vi "Run.vi"(8 "error in (no error)":errorcluster, 9 "Penalty":dbl, 10 "Maze (0: Empty, -1: Enemy. 1: Teammate":i32[][](array[numeric]), 11 "Runner in":refnum<class "Circle the Wagons.lvclass">) -> (0 "error out":errorcluster, 1 "Direction":T1, 2 "Action":T2, 3 "Runner out":refnum<class "Circle the Wagons.lvclass">, 4 "Replicated":refnum<class "Square.lvclass">)   [LabVIEW 2015, in "Circle the Wagons.lvclass"]
uses:
  Circle the Wagons.lvclass
  Type Defs/Action Enum.ctl
  Type Defs/Direction Enum.ctl
  Square/Square.lvclass
  DVR Cluster.ctl
  Circle the Wagons.lvclass/Circle the Wagons.ctl
  SubVIs/Read-Only Globals.vi
  Type Defs/SB Type Defs.lvlib
panel:
  # "NOTICE - YOU MUST NOT REMOVE THIS NOTICE. PER THE FOLLOWING LICENSE, YOU MAY REPRODUCE THIS SOFTWARE PROVIDED YOU FOLLOW THE TERMS\nOF THE LICENSE.\n\n---BEGIN BSD LICENSE (http://opensource.org/licenses/BSD-2-Clause)---\nCopyright (c) 2015, Endigit, Inc. <robert@endigit.com>\nAll rights reserved.\n\nRedistribution and use in source and binary forms, with or without modification, are permitted provided that the following conditions are met:\n\n1. Redistributions of source code must retain the above copyright notice, this list of conditions and the following disclaimer.\n\n2. Redistributions in binary form must reproduce the above copyright notice, this list of conditions and the following disclaimer in the documentation and/or other \nmaterials provided with the distribution.\n\nTHIS SOFTWARE IS PROVIDED BY THE COPYRIGHT HOLDERS AND CONTRIBUTORS \"AS IS\" AND ANY EXPRESS OR IMPLIED WARRANTIES, INCLUDING, BUT NOT \nLIMITED TO, THE IMPLIED WARRANTIES OF MERCHANTABILITY AND FITNESS FOR A PARTICULAR PURPOSE ARE DISCLAIMED. IN NO EVENT SHALL THE COPYRIGHT \nHOLDER OR CONTRIBUTORS BE LIABLE FOR ANY DIRECT, INDIRECT, INCIDENTAL, SPECIAL, EXEMPLARY, OR CONSEQUENTIAL DAMAGES (INCLUDING, BUT NOT \nLIMITED TO, PROCUREMENT OF SUBSTITUTE GOODS OR SERVICES; LOSS OF USE, DATA, OR PROFITS; OR BUSINESS INTERRUPTION) HOWEVER CAUSED AND ON \nANY THEORY OF LIABILITY, WHETHER IN CONTRACT, STRICT LIABILITY, OR TORT (INCLUDING NEGLIGENCE OR OTHERWISE) ARISING IN ANY WAY OUT OF THE USE \nOF THIS SOFTWARE, EVEN IF ADVISED OF THE POSSIBILITY OF SUCH DAMAGE.\n---END BSD LICENSE---"
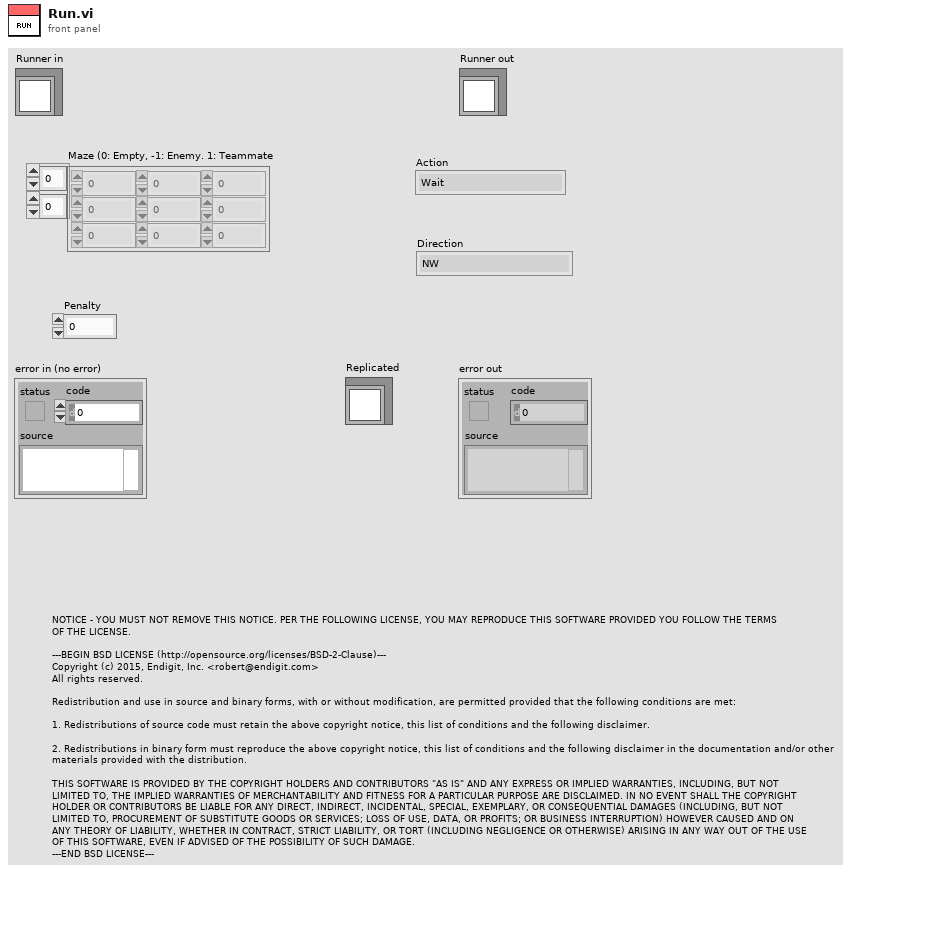
[diagram p1: front panel]
types:
  T1 = typedef "SB Type Defs.lvlib/Direction Enum.ctl" = enum16{"NW", "N", "NE", "E", "SE", "S", "SW", "W"}
  T2 = typedef "SB Type Defs.lvlib/Action Enum.ctl" = enum16{"Wait", "Move", "Attack", "Replicate"}
  T3 = typedef "Circle the Wagons.lvclass/DVR Cluster.ctl" = cluster{"Stage":i32}
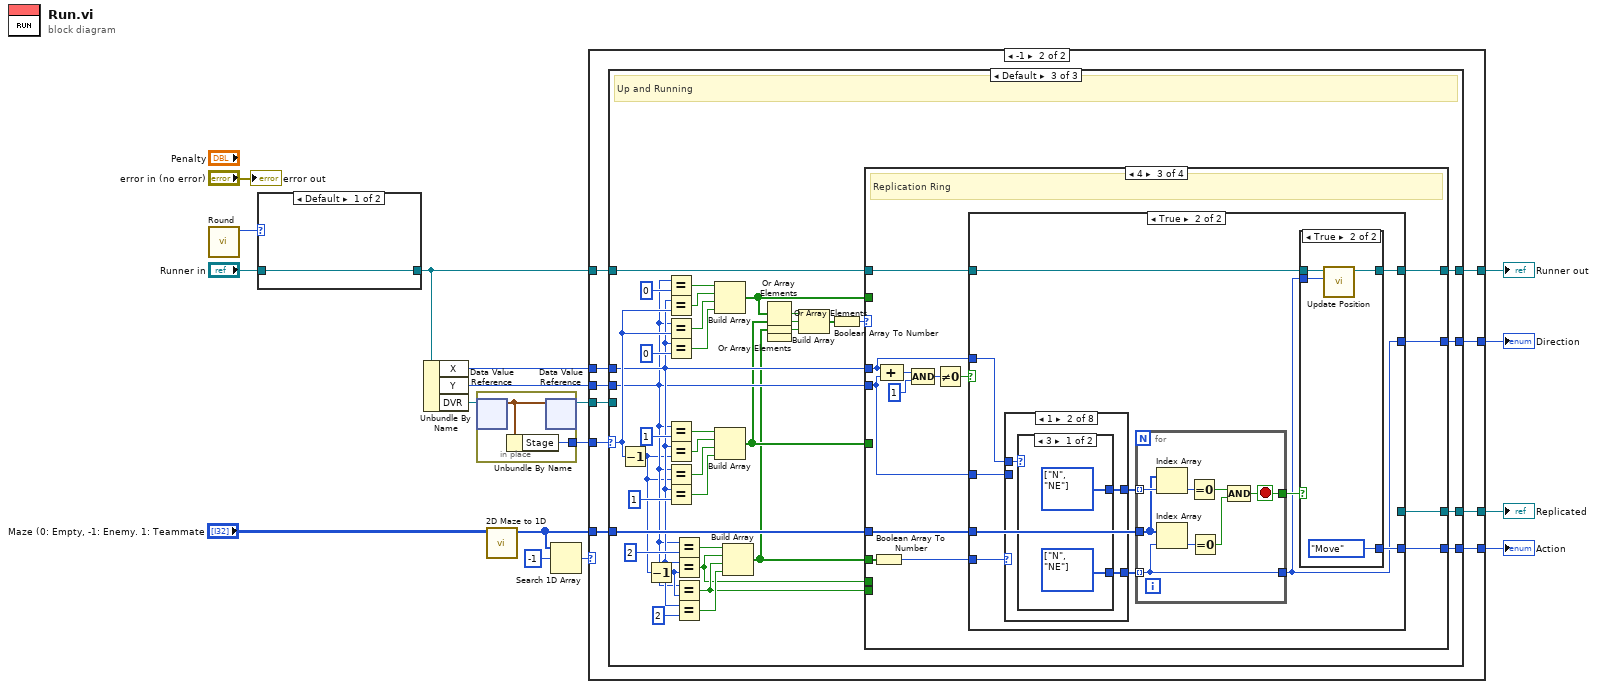
[diagram p0: block diagram]
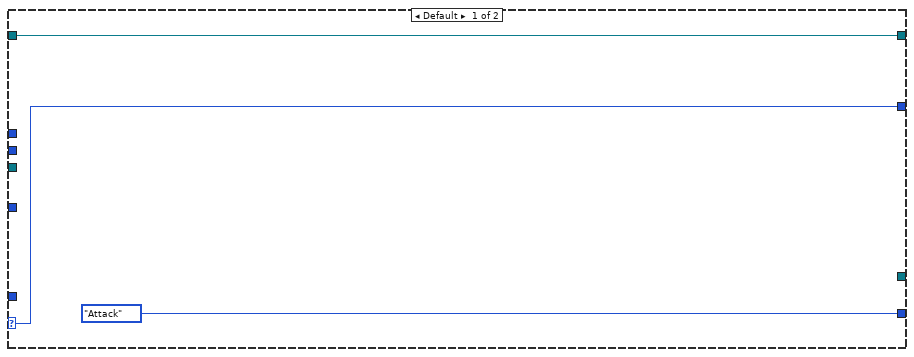
[diagram p2: hidden frame]
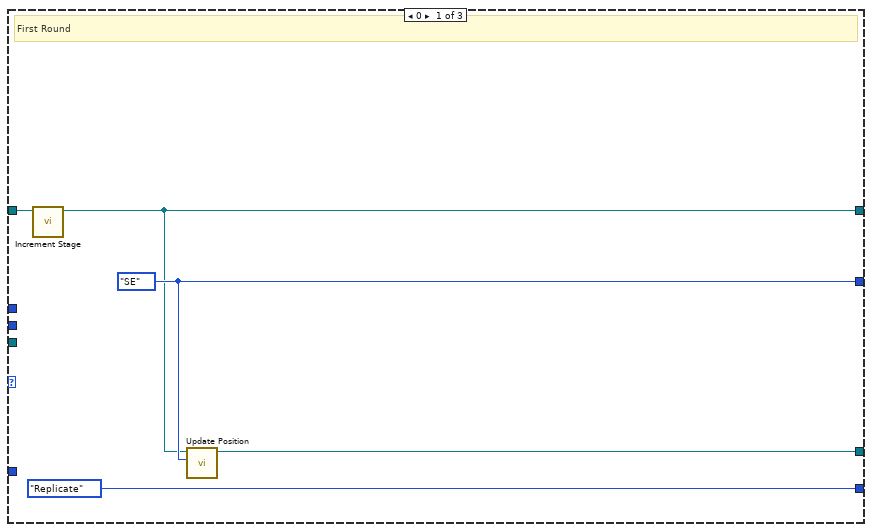
[diagram p3: hidden frame]
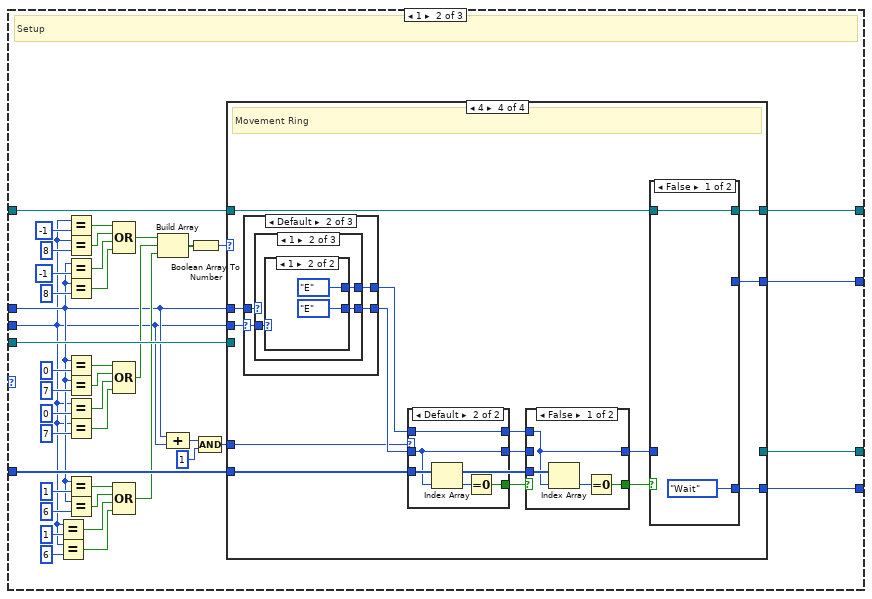
[diagram p4: hidden frame]
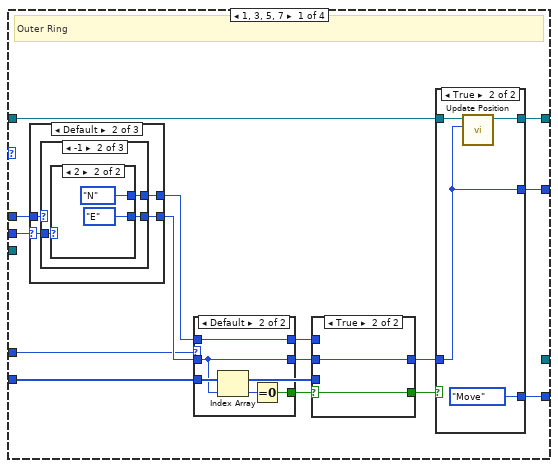
[diagram p5: hidden frame]
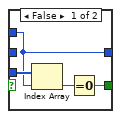
[diagram p6: hidden frame]
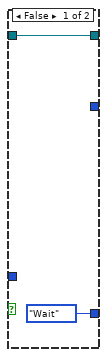
[diagram p8: hidden frame]
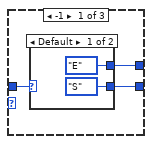
[diagram p9: hidden frame]
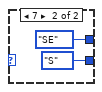
[diagram p10: hidden frame]
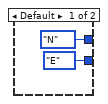
[diagram p12: hidden frame]
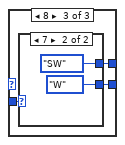
[diagram p13: hidden frame]
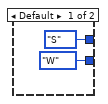
[diagram p14: hidden frame]
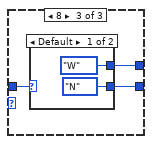
[diagram p15: hidden frame]
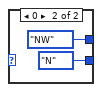
[diagram p16: hidden frame]
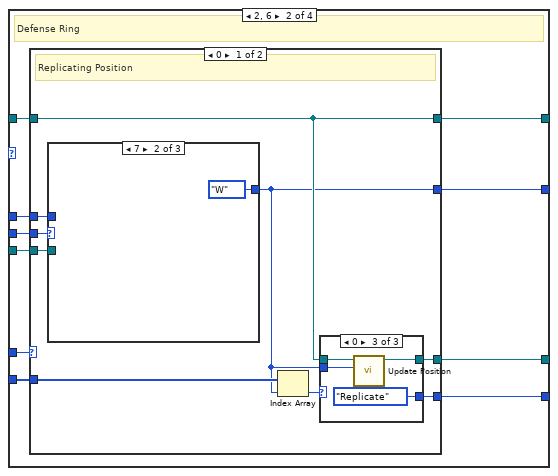
[diagram p17: hidden frame]
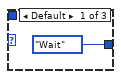
[diagram p18: hidden frame]
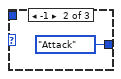
[diagram p19: hidden frame]
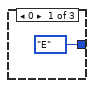
[diagram p20: hidden frame]
diagram:
  n1 = call "Round.vi"() -> ("Round"=w16:i32)  [unwired: 11 in]
  n2 = case shown="Default" w16 {
    tunnel: "Runner in" -> [w18 w21]
    tunnel: [w18 w19] -> w13
    frame Default {
    }
    frame 0 {
      n3 = New Data Value Reference(data value=T3 {"Stage"=0} ("DVR Cluster")) -> (data value reference=w20:refnum<data-value>)  [unwired: 1 in, 1 out]
      n4 = Bundle By Name(cluster=w21, "DVR"=w20) -> (w19:refnum<class "Circle the Wagons.lvclass">)
    }
  }
  n5 = Unbundle By Name(w13) -> ("X"=w11:i32, "Y"=w10:i32, "DVR"=w14:refnum<data-value>)
  n6 = in-place {
    in-place-border: [w23] -> w9
    n7 = in-place-dvr #1(w14) -> (w24:T3)  [unwired: 1 out]
    n8 = Unbundle By Name(w24) -> ("Stage"=w23:i32)
    n9 = in-place-dvr #1(w24) -> (w4:refnum<data-value>)  [unwired: 1 out]
  }
  n10 = call "2D Maze to 1D.vi"("Maze (0: Empty, -1: Enemy. >0: Teammate"="Maze (0: Empty, -1: Enemy. 1: Teammate") -> ("1D Maze"=w2:i32[])  [unwired: 10 in]
  n11 = Search 1D Array(1D array=w2, element=-1) -> (index of element=w1:i32)  [unwired: 1 in]
  n12 = case shown="-1" w1 {
    selector: w1 -> [w25 _]
    tunnel: w13 -> [w27 w37]
    tunnel: [w27 w36] -> w12
    tunnel: w11 -> [_ w35]
    tunnel: w10 -> [_ w34]
    tunnel: w9 -> [_ w33]
    tunnel: [w25 w32] -> w8
    tunnel: [Action_Enum."Attack" ("Action") w31] -> w7
    tunnel: [_ w30] -> w6
    tunnel: w4 -> [_ w29]
    tunnel: w2 -> [_ w28]
    frame Default {
    }
    frame -1 {
      n13 = case shown="Default" w33 {
        selector: w33 -> [_ _ w369]
        tunnel: w37 -> [w41 w82 w381]
        tunnel: [w38 w77 w377] -> w36
        tunnel: w35 -> [_ w45 w355]
        tunnel: w34 -> [_ w44 w354]
        tunnel: w28 -> [_ w83 w382]
        tunnel: [w40 w81 w380] -> w32
        tunnel: [Action_Enum."Replicate" ("Action") w80 w379] -> w31
        tunnel: w29 -> [_ w79 _]
        tunnel: [w39 w78 w378] -> w30
        frame 0 {
          w40 = Direction_Enum."SE" ("Direction")
          # "First Round"
          n14 = call "Increment Stage.vi"("Circle the Wagons in"=w41) -> ("Circle the Wagons out"=w38:refnum<class "Circle the Wagons.lvclass">)  [unwired: 10 in]
          n15 = call "Update Position.vi"("Direction"=w40, "Circle the Wagons in"=w38) -> ("Circle the Wagons out"=w39:refnum<class "Circle the Wagons.lvclass">)  [unwired: 9 in]
        }
        frame 1 {
          # "Setup"
          n16 = Equal?(x=w44, y=1) -> (x = y?=w56:bool)
          n17 = Equal?(x=w44, y=6) -> (x = y?=w55:bool)
          n18 = Equal?(x=w44, y=-1) -> (x = y?=w65:bool)
          n19 = Equal?(x=w44, y=8) -> (x = y?=w66:bool)
          n20 = Equal?(x=w45, y=-1) -> (x = y?=w68:bool)
          n21 = Equal?(x=w45, y=8) -> (x = y?=w67:bool)
          n22 = Equal?(x=w45, y=0) -> (x = y?=w72:bool)
          n23 = Equal?(x=w45, y=7) -> (x = y?=w71:bool)
          n24 = Equal?(x=w44, y=0) -> (x = y?=w69:bool)
          n25 = Equal?(x=w44, y=7) -> (x = y?=w70:bool)
          n26 = Equal?(x=w45, y=1) -> (x = y?=w53:bool)
          n27 = Equal?(x=w45, y=6) -> (x = y?=w54:bool)
          n28 = Compound Arithmetic op=OR(w65, w66, w68, w67) -> (w60:bool)
          n29 = Compound Arithmetic op=OR(w72, w71, w69, w70) -> (w59:bool)
          n30 = Compound Arithmetic op=OR(w53, w54, w56, w55) -> (w48:bool)
          n31 = Build Array(w60, w59, w48) -> (w58:bool[])
          n32 = Compound Arithmetic op=ADD(w45, w44) -> (w46:i32)
          n33 = Boolean Array To Number(Boolean array=w58) -> (number=w57:u32)
          n34 = Compound Arithmetic op=AND(w46, 1 ("value")) -> (w43:i32)
          n35 = case shown="4" w57 {
            tunnel: w83 -> [w92 w152 w221 w288]
            tunnel: w82 -> [w98 w159 w228 w294]
            tunnel: [w97 w158 w227 w293] -> w81
            tunnel: [w96 w157 w226 w292] -> w80
            tunnel: w79 -> [_ w150 _ _]
            tunnel: [_ w156 w225 _] -> w78
            tunnel: [w95 w155 w224 w291] -> w77
            tunnel: w45 -> [w94 w154 w223 w290]
            tunnel: w44 -> [w93 w153 w222 w289]
            tunnel: w43 -> [w84 w151 w220 w280]
            frame 1, 3, 5, 7 {
              # "Outer Ring"
              n36 = case shown="Default" w93 {
                selector: w93 -> [_ w125 _]
                tunnel: w94 -> [w119 w127 w144]
                tunnel: [w120 w128 w145] -> w90
                tunnel: [w118 w126 w143] -> w91
                frame -1 {
                  n37 = case shown="Default" w119 {
                    tunnel: [Direction_Enum."E" ("Direction") Direction_Enum."SE" ("Direction")] -> w120
                    tunnel: [Direction_Enum."S" ("Direction") Direction_Enum."S" ("Direction")] -> w118
                    frame Default {
                    }
                    frame 7 {
                    }
                  }
                }
                frame Default {
                  n38 = case shown="-1" w127 {
                    tunnel: [_ w131 w138] -> w128
                    tunnel: [_ w130 w137] -> w126
                    tunnel: w125 -> [_ w129 w136]
                    frame Default {
                    }
                    frame -1 {
                      n39 = case shown="2" w129 {
                        tunnel: [Direction_Enum."N" ("Direction") Direction_Enum."N" ("Direction")] -> w131
                        tunnel: [Direction_Enum."E" ("Direction") Direction_Enum."E" ("Direction")] -> w130
                        frame Default {
                        }
                        frame 2 {
                        }
                      }
                    }
                    frame 8 {
                      n40 = case shown="7" w136 {
                        tunnel: [Direction_Enum."S" ("Direction") Direction_Enum."SW" ("Direction")] -> w138
                        tunnel: [Direction_Enum."W" ("Direction") Direction_Enum."W" ("Direction")] -> w137
                        frame Default {
                        }
                        frame 7 {
                        }
                      }
                    }
                  }
                }
                frame 8 {
                  n41 = case shown="Default" w144 {
                    tunnel: [Direction_Enum."W" ("Direction") Direction_Enum."NW" ("Direction")] -> w145
                    tunnel: [Direction_Enum."N" ("Direction") Direction_Enum."N" ("Direction")] -> w143
                    frame Default {
                    }
                    frame 0 {
                    }
                  }
                }
              }
              n42 = case shown="Default" w84 {
                tunnel: w92 -> [_ w111]
                tunnel: w91 -> [w105 w107]
                tunnel: [_ w109] -> w89
                tunnel: w90 -> [w106 w108]
                tunnel: [w106 w108] -> w88
                tunnel: [w105 w107] -> w87
                frame 0 {
                }
                frame Default {
                  n43 = Index Array(array=w111, index=w107) -> (element=w110:i32)
                  n44 = Equal To 0?(x=w110) -> (x = 0?=w109:bool)
                }
              }
              n45 = case shown="True" w89 {
                selector: w89 -> [_ w103]
                tunnel: w88 -> [w99 _]
                tunnel: w87 -> [_ w104]
                tunnel: [w99 w104] -> w85
                tunnel: [w100 w103] -> w86
                tunnel: w92 -> [w102 _]
                frame False {
                  n46 = Index Array(array=w102, index=w99) -> (element=w101:i32)
                  n47 = Equal To 0?(x=w101) -> (x = 0?=w100:bool)
                }
                frame True {
                }
              }
              n48 = case shown="True" w86 {
                tunnel: w98 -> [w113 w117]
                tunnel: [w113 w116] -> w95
                tunnel: [Action_Enum."Wait" ("Action") Action_Enum."Move" ("Action")] -> w96
                tunnel: [_ w114] -> w97
                tunnel: w85 -> [_ w114]
                frame False {
                }
                frame True {
                  n49 = call "Update Position.vi"("Direction"=w114, "Circle the Wagons in"=w117) -> ("Circle the Wagons out"=w116:refnum<class "Circle the Wagons.lvclass">)  [unwired: 9 in]
                }
              }
            }
            frame 2, 6 {
              # "Defense Ring"
              n50 = case shown="0" w151 {
                tunnel: w154 -> [w167 w200]
                tunnel: w153 -> [w166 w199]
                tunnel: w152 -> [w168 w196]
                tunnel: w159 -> [w162 w198]
                tunnel: [w161 w202] -> w158
                tunnel: [w164 w201] -> w157
                tunnel: [w163 _] -> w156
                tunnel: [w162 w197] -> w155
                tunnel: w150 -> [w160 _]
                frame 0 {
                  # "Replicating Position"
                  n51 = case shown="7" w166 {
                    selector: w166 -> [_ _ w178]
                    tunnel: w167 -> [_ _ w180]
                    tunnel: [Direction_Enum."E" ("Direction") Direction_Enum."W" ("Direction") w179] -> w161
                    tunnel: w160 -> [_ _ w177]
                    frame 0 {
                    }
                    frame 7 {
                    }
                    frame Default {
                      n52 = case shown="7" w180 {
                        tunnel: [_ Direction_Enum."N" ("Direction") Direction_Enum."S" ("Direction")] -> w179
                        tunnel: w178 -> [_ w182 _]
                        tunnel: w177 -> [_ w181 _]
                        frame Default {
                        }
                        frame 0 {
                          n53 = case shown="2" w182 {
                            tunnel: w181 -> [_ w184]
                            frame Default {
                            }
                            frame 2 {
                              n54 = in-place {
                                n55 = in-place-dvr #2(w184) -> (w187:T3)  [unwired: 1 out]
                                n56 = Bundle By Name(cluster=w187, "Stage"=7) -> (w185:T3)
                                n57 = in-place-dvr #2(w185) -> ()  [unwired: 2 out]
                              }
                            }
                          }
                        }
                        frame 7 {
                        }
                      }
                    }
                  }
                  n58 = Index Array(array=w168, index=w161) -> (element=w165:i32)
                  n59 = case shown="0" w165 {
                    tunnel: [Action_Enum."Wait" ("Action") Action_Enum."Attack" ("Action") Action_Enum."Replicate" ("Action")] -> w164
                    tunnel: [_ _ w173] -> w163
                    tunnel: w161 -> [_ _ w172]
                    tunnel: w162 -> [_ _ w171]
                    frame Default {
                    }
                    frame -1 {
                    }
                    frame 0 {
                      n60 = call "Update Position.vi"("Direction"=w172, "Circle the Wagons in"=w171) -> ("Circle the Wagons out"=w173:refnum<class "Circle the Wagons.lvclass">)  [unwired: 9 in]
                    }
                  }
                }
                frame Default {
                  # "Non-replicating Position"
                  n61 = case shown="0" w200 {
                    tunnel: [Direction_Enum."W" ("Direction") Direction_Enum."E" ("Direction") w215] -> w194
                    tunnel: [Direction_Enum."NW" ("Direction") Direction_Enum."SE" ("Direction") w214] -> w189
                    tunnel: w199 -> [_ _ w213]
                    frame 0 {
                    }
                    frame 7 {
                    }
                    frame Default {
                      n62 = case shown="7" w213 {
                        tunnel: [_ Direction_Enum."N" ("Direction") Direction_Enum."S" ("Direction")] -> w215
                        tunnel: [_ Direction_Enum."NE" ("Direction") Direction_Enum."SW" ("Direction")] -> w214
                        frame Default {
                        }
                        frame 0 {
                        }
                        frame 7 {
                        }
                      }
                    }
                  }
                  n63 = Index Array(array=w196, index=w189) -> (element=w195:i32)
                  n64 = Index Array(array=w196, index=w194) -> (element=w193:i32)
                  n65 = Equal To 0?(x=w193) -> (x = 0?=w191:bool)
                  n66 = Equal To 0?(x=w195) -> (x = 0?=w192:bool)
                  n67 = Compound Arithmetic op=AND(w192, w191) -> (w190:bool)
                  n68 = case shown="True" w190 {
                    tunnel: w198 -> [w204 w208]
                    tunnel: [w204 w207] -> w197
                    tunnel: [Action_Enum."Wait" ("Action") Action_Enum."Move" ("Action")] -> w201
                    tunnel: [_ w205] -> w202
                    tunnel: w189 -> [_ w205]
                    frame False {
                    }
                    frame True {
                      n69 = call "Update Position.vi"("Direction"=w205, "Circle the Wagons in"=w208) -> ("Circle the Wagons out"=w207:refnum<class "Circle the Wagons.lvclass">)  [unwired: 9 in]
                    }
                  }
                }
              }
            }
            frame Default {
              # "Replication Ring"
              n70 = case shown="0" w220 {
                tunnel: w223 -> [w232 w260]
                tunnel: w222 -> [w231 w259]
                tunnel: w221 -> [w236 w256]
                tunnel: w228 -> [w229 w258]
                tunnel: [w230 w262] -> w227
                tunnel: [w234 w261] -> w226
                tunnel: [w233 _] -> w225
                tunnel: [w229 w257] -> w224
                frame 0 {
                  # "Replicating Position"
                  n71 = case shown="2" w231 {
                    tunnel: w232 -> [_ _ w246]
                    tunnel: [Direction_Enum."E" ("Direction") Direction_Enum."W" ("Direction") w245] -> w230
                    frame 2 {
                    }
                    frame 5 {
                    }
                    frame Default {
                      n72 = case shown="5" w246 {
                        tunnel: [_ Direction_Enum."N" ("Direction") Direction_Enum."S" ("Direction")] -> w245
                        frame Default {
                        }
                        frame 2 {
                        }
                        frame 5 {
                        }
                      }
                    }
                  }
                  n73 = Index Array(array=w236, index=w230) -> (element=w235:i32)
                  n74 = case shown="0" w235 {
                    tunnel: [Action_Enum."Wait" ("Action") Action_Enum."Attack" ("Action") Action_Enum."Replicate" ("Action")] -> w234
                    tunnel: [_ _ w241] -> w233
                    tunnel: w230 -> [_ _ w240]
                    tunnel: w229 -> [_ _ w239]
                    frame Default {
                    }
                    frame -1 {
                    }
                    frame 0 {
                      n75 = call "Update Position.vi"("Direction"=w240, "Circle the Wagons in"=w239) -> ("Circle the Wagons out"=w241:refnum<class "Circle the Wagons.lvclass">)  [unwired: 9 in]
                    }
                  }
                }
                frame Default {
                  # "Non-replicating Position"
                  n76 = case shown="Default" w260 {
                    tunnel: [Direction_Enum."W" ("Direction") Direction_Enum."E" ("Direction") w275] -> w254
                    tunnel: [Direction_Enum."NW" ("Direction") Direction_Enum."SE" ("Direction") w274] -> w249
                    tunnel: w259 -> [_ _ w273]
                    frame 2 {
                    }
                    frame 5 {
                    }
                    frame Default {
                      n77 = case shown="2" w273 {
                        tunnel: [_ Direction_Enum."N" ("Direction") Direction_Enum."S" ("Direction")] -> w275
                        tunnel: [_ Direction_Enum."NE" ("Direction") Direction_Enum."SW" ("Direction")] -> w274
                        frame Default {
                        }
                        frame 2 {
                        }
                        frame 5 {
                        }
                      }
                    }
                  }
                  n78 = Index Array(array=w256, index=w249) -> (element=w255:i32)
                  n79 = Index Array(array=w256, index=w254) -> (element=w253:i32)
                  n80 = Equal To 0?(x=w253) -> (x = 0?=w251:bool)
                  n81 = Equal To 0?(x=w255) -> (x = 0?=w252:bool)
                  n82 = Compound Arithmetic op=AND(w252, w251) -> (w250:bool)
                  n83 = case shown="True" w250 {
                    tunnel: w258 -> [w264 w268]
                    tunnel: [w264 w267] -> w257
                    tunnel: [Action_Enum."Wait" ("Action") Action_Enum."Move" ("Action")] -> w261
                    tunnel: [_ w265] -> w262
                    tunnel: w249 -> [_ w265]
                    frame False {
                    }
                    frame True {
                      n84 = call "Update Position.vi"("Direction"=w265, "Circle the Wagons in"=w268) -> ("Circle the Wagons out"=w267:refnum<class "Circle the Wagons.lvclass">)  [unwired: 9 in]
                    }
                  }
                }
              }
            }
            frame 4 {
              # "Movement Ring"
              n85 = case shown="Default" w289 {
                selector: w289 -> [_ w321 _]
                tunnel: w290 -> [w315 w323 w340]
                tunnel: [w316 w324 w341] -> w286
                tunnel: [w314 w322 w339] -> w287
                frame 1 {
                  n86 = case shown="Default" w315 {
                    tunnel: [Direction_Enum."E" ("Direction") Direction_Enum."S" ("Direction")] -> w316
                    tunnel: [Direction_Enum."S" ("Direction") Direction_Enum."S" ("Direction")] -> w314
                    frame Default {
                    }
                    frame 6 {
                    }
                  }
                }
                frame Default {
                  n87 = case shown="1" w323 {
                    tunnel: [_ w327 w334] -> w324
                    tunnel: [_ w326 w333] -> w322
                    tunnel: w321 -> [_ w325 w332]
                    frame Default {
                    }
                    frame 1 {
                      n88 = case shown="1" w325 {
                        tunnel: [Direction_Enum."N" ("Direction") Direction_Enum."E" ("Direction")] -> w327
                        tunnel: [Direction_Enum."E" ("Direction") Direction_Enum."E" ("Direction")] -> w326
                        frame Default {
                        }
                        frame 1 {
                        }
                      }
                    }
                    frame 6 {
                      n89 = case shown="Default" w332 {
                        tunnel: [Direction_Enum."S" ("Direction") Direction_Enum."W" ("Direction")] -> w334
                        tunnel: [Direction_Enum."W" ("Direction") Direction_Enum."W" ("Direction")] -> w333
                        frame Default {
                        }
                        frame 6 {
                        }
                      }
                    }
                  }
                }
                frame 6 {
                  n90 = case shown="1" w340 {
                    tunnel: [Direction_Enum."W" ("Direction") Direction_Enum."N" ("Direction")] -> w341
                    tunnel: [Direction_Enum."N" ("Direction") Direction_Enum."N" ("Direction")] -> w339
                    frame Default {
                    }
                    frame 1 {
                    }
                  }
                }
              }
              n91 = case shown="Default" w280 {
                tunnel: w288 -> [_ w307]
                tunnel: w287 -> [w301 w303]
                tunnel: [_ w305] -> w285
                tunnel: w286 -> [w302 w304]
                tunnel: [w302 w304] -> w284
                tunnel: [w301 w303] -> w283
                frame 0 {
                }
                frame Default {
                  n92 = Index Array(array=w307, index=w303) -> (element=w306:i32)
                  n93 = Equal To 0?(x=w306) -> (x = 0?=w305:bool)
                }
              }
              n94 = case shown="False" w285 {
                selector: w285 -> [_ w299]
                tunnel: w284 -> [w295 _]
                tunnel: w283 -> [_ w300]
                tunnel: [w295 w300] -> w281
                tunnel: [w296 w299] -> w282
                tunnel: w288 -> [w298 _]
                frame False {
                  n95 = Index Array(array=w298, index=w295) -> (element=w297:i32)
                  n96 = Equal To 0?(x=w297) -> (x = 0?=w296:bool)
                }
                frame True {
                }
              }
              n97 = case shown="False" w282 {
                tunnel: w294 -> [w309 w313]
                tunnel: [w309 w312] -> w291
                tunnel: [Action_Enum."Wait" ("Action") Action_Enum."Move" ("Action")] -> w292
                tunnel: [_ w310] -> w293
                tunnel: w281 -> [_ w310]
                frame False {
                }
                frame True {
                  n98 = call "Update Position.vi"("Direction"=w310, "Circle the Wagons in"=w313) -> ("Circle the Wagons out"=w312:refnum<class "Circle the Wagons.lvclass">)  [unwired: 9 in]
                }
              }
            }
          }
        }
        frame Default {
          # "Up and Running"
          n99 = Decrement(x=w369) -> (x-1=w352:i32)
          n100 = Decrement(x=w352) -> (x-1=w360:i32)
          n101 = Equal?(x=w354, y=0) -> (x = y?=w373:bool)
          n102 = Equal?(x=w355, y=w369) -> (x = y?=w374:bool)
          n103 = Equal?(x=w354, y=w369) -> (x = y?=w376:bool)
          n104 = Equal?(x=w355, y=0) -> (x = y?=w375:bool)
          n105 = Equal?(x=w354, y=1) -> (x = y?=w364:bool)
          n106 = Equal?(x=w355, y=w352) -> (x = y?=w363:bool)
          n107 = Equal?(x=w354, y=w352) -> (x = y?=w348:bool)
          n108 = Equal?(x=w355, y=1) -> (x = y?=w362:bool)
          n109 = Equal?(x=w354, y=2) -> (x = y?=w358:bool)
          n110 = Equal?(x=w355, y=w360) -> (x = y?=w346:bool)
          n111 = Equal?(x=w354, y=w360) -> (x = y?=w347:bool)
          n112 = Equal?(x=w355, y=2) -> (x = y?=w359:bool)
          n113 = Build Array(w373, w374, w376, w375) -> (w351:bool[])
          n114 = Build Array(w364, w363, w348, w362) -> (w350:bool[])
          n115 = Build Array(w358, w346, w347, w359) -> (w349:bool[])
          n116 = Or Array Elements(Boolean array=w351) -> (logical OR=w367:bool)
          n117 = Or Array Elements(Boolean array=w350) -> (logical OR=w361:bool)
          n118 = Or Array Elements(Boolean array=w349) -> (logical OR=w353:bool)
          n119 = Build Array(w367, w361, w353) -> (w371:bool[])
          n120 = Boolean Array To Number(Boolean array=w371) -> (number=w370:u32)
          n121 = case shown="4" w370 {
            tunnel: w382 -> [_ w396 w496 w580]
            tunnel: w381 -> [w386 w412 w503 w584]
            tunnel: [w383 w402 w502 w581] -> w380
            tunnel: [Action_Enum."Attack" ("Action") w411 w501 w583] -> w379
            tunnel: [_ _ w493 _] -> w378
            tunnel: [w386 w413 w504 w582] -> w377
            tunnel: w355 -> [_ w401 w492 w577]
            tunnel: w354 -> [_ w397 w491 w576]
            tunnel: w351 -> [w385 _ _ _]
            tunnel: w350 -> [_ w410 _ _]
            tunnel: w349 -> [_ _ w495 _]
            tunnel: w347 -> [_ w400 _ _]
            tunnel: w346 -> [_ w398 _ _]
            frame 1, 3, 5, 7 {
              # "Defense Ring"
              n122 = Boolean Array To Number(Boolean array=w385) -> (number=w384:u32)
              n123 = case shown="12" w384 {
                tunnel: [Direction_Enum."NW" ("Direction") Direction_Enum."N" ("Direction") Direction_Enum."NE" ("Direction") Direction_Enum."E" ("Direction") Direction_Enum."SE" ("Direction") Direction_Enum."S" ("Direction") Direction_Enum."SW" ("Direction") Direction_Enum."W" ("Direction") _] -> w383
                frame 9 {
                }
                frame 1 {
                }
                frame 3 {
                }
                frame 2 {
                }
                frame 6 {
                }
                frame 4 {
                }
                frame 12 {
                }
                frame 8 {
                }
                frame Default {
                }
              }
            }
            frame 2, 6 {
              # "Movement Ring"
              n124 = Boolean Array To Number(Boolean array=w410) -> (number=w409:u32)
              n125 = Compound Arithmetic op=ADD(w401, w397) -> (w408:i32)
              n126 = Compound Arithmetic op=AND(w408, 1 ("value")) -> (w406:i32)
              n127 = Not Equal To 0?(x=w406) -> (x != 0?=w405:bool)
              n128 = case shown="4" w409 {
                tunnel: w405 -> [_ _ w432 _ w444 _ w465 _ w481]
                tunnel: [_ w429 w431 w439 w443 w454 w458 w474 w480] -> w404
                tunnel: w401 -> [_ _ w430 _ _ _ _ _ _]
                tunnel: w400 -> [_ _ _ _ w442 _ _ _ _]
                tunnel: [_ _ _ _ w441 _ _ _ _] -> w399
                tunnel: w398 -> [_ _ _ _ _ _ w464 _ _]
                tunnel: w397 -> [_ _ _ _ _ _ _ _ w479]
                tunnel: w396 -> [_ _ _ _ w440 _ w463 _ w478]
                frame Default {
                }
                frame 9 {
                  w429 = T1[] [enum."NW"] items=["NW", "N", "NE", "E", "SE", "S", "SW", "W"]
                }
                frame 1 {
                  n129 = case shown="3" w430 {
                    tunnel: w432 -> [_ _ w438]
                    tunnel: [w433 w434 w435] -> w431
                    frame 2 {
                      w433 = T1[] [enum."NE", enum."N", enum."NW", enum."W"] items=["NW", "N", "NE", "E", "SE", "S", "SW", "W"]
                    }
                    frame 3 {
                      w434 = T1[] [enum."W"] items=["NW", "N", "NE", "E", "SE", "S", "SW", "W"]
                    }
                    frame Default {
                      w436 = T1[] [enum."N", enum."E"] items=["NW", "N", "NE", "E", "SE", "S", "SW", "W"]
                      w437 = T1[] [enum."N", enum."S", enum."E"] items=["NW", "N", "NE", "E", "SE", "S", "SW", "W"]
                      n130 = Select(t=w437, s=w438, f=w436) -> (s? t:f=w435:T1[])
                    }
                  }
                }
                frame 3 {
                  w439 = T1[] [enum."N", enum."E", enum."NE", enum."S"] items=["NW", "N", "NE", "E", "SE", "S", "SW", "W"]
                }
                frame 2 {
                  n131 = case shown="True" w442 {
                    tunnel: w444 -> [w448 _]
                    tunnel: [w447 w450] -> w443
                    tunnel: [_ w449] -> w441
                    tunnel: w440 -> [_ w453]
                    frame False {
                      w445 = T1[] [enum."E", enum."S"] items=["NW", "N", "NE", "E", "SE", "S", "SW", "W"]
                      w446 = T1[] [enum."E", enum."W", enum."S"] items=["NW", "N", "NE", "E", "SE", "S", "SW", "W"]
                      n132 = Select(t=w446, s=w448, f=w445) -> (s? t:f=w447:T1[])
                    }
                    frame True {
                      w450 = T1[] [enum."E", enum."SE", enum."S"] items=["NW", "N", "NE", "E", "SE", "S", "SW", "W"]
                      n133 = Index Array(array=w453, index=Direction_Enum."SW" ("Direction")) -> (element=w451:i32)
                      n134 = Greater Than 0?(x=w451) -> (x > 0?=w449:bool)
                    }
                  }
                }
                frame 6 {
                  w454 = T1[] [enum."SE"] items=["NW", "N", "NE", "E", "SE", "S", "SW", "W"]
                }
                frame 4 {
                  w455 = T1[] [enum."E"] items=["NW", "N", "NE", "E", "SE", "S", "SW", "W"]
                  w456 = T1[] [] items=["NW", "N", "NE", "E", "SE", "S", "SW", "W"]
                  n135 = case shown="False" w464 {
                    tunnel: w465 -> [w469 w473]
                    tunnel: [w466 w470] -> w459
                    frame True {
                      w467 = T1[] [enum."S", enum."SE"] items=["NW", "N", "NE", "E", "SE", "S", "SW", "W"]
                      w468 = T1[] [enum."S", enum."SE", enum."N"] items=["NW", "N", "NE", "E", "SE", "S", "SW", "W"]
                      n136 = Select(t=w468, s=w469, f=w467) -> (s? t:f=w466:T1[])
                    }
                    frame False {
                      w471 = T1[] [enum."S", enum."E"] items=["NW", "N", "NE", "E", "SE", "S", "SW", "W"]
                      w472 = T1[] [enum."S", enum."N", enum."E"] items=["NW", "N", "NE", "E", "SE", "S", "SW", "W"]
                      n137 = Select(t=w472, s=w473, f=w471) -> (s? t:f=w470:T1[])
                    }
                  }
                  n138 = Index Array(array=w463, index=Direction_Enum."NE" ("Direction")) -> (element=w461:i32)
                  n139 = Equal To 0?(x=w461) -> (x = 0?=w460:bool)
                  n140 = Select(t=w455, s=w460, f=w456) -> (s? t:f=w457:T1[])
                  n141 = Build Array (concatenate)(w459, w457) -> (w458:T1[])
                }
                frame 12 {
                  w474 = T1[] [enum."W", enum."S", enum."SW", enum."E"] items=["NW", "N", "NE", "E", "SE", "S", "SW", "W"]
                }
                frame 8 {
                  n142 = Index Array(array=w478, index=Direction_Enum."NE" ("Direction")) -> (element=w476:i32)
                  n143 = Equal To 0?(x=w476) -> (x = 0?=w475:bool)
                  n144 = case shown="2" w479 {
                    tunnel: w481 -> [_ _ w490]
                    tunnel: [w485 w486 w487] -> w480
                    tunnel: w475 -> [w483 _ _]
                    frame 2 {
                      w482 = T1[] [enum."SW", enum."W", enum."NW"] items=["NW", "N", "NE", "E", "SE", "S", "SW", "W"]
                      w484 = T1[] [enum."SW", enum."W", enum."NW", enum."N"] items=["NW", "N", "NE", "E", "SE", "S", "SW", "W"]
                      n145 = Select(t=w484, s=w483, f=w482) -> (s? t:f=w485:T1[])
                    }
                    frame 3 {
                      w486 = T1[] [enum."N"] items=["NW", "N", "NE", "E", "SE", "S", "SW", "W"]
                    }
                    frame Default {
                      w488 = T1[] [enum."W", enum."S"] items=["NW", "N", "NE", "E", "SE", "S", "SW", "W"]
                      w489 = T1[] [enum."W", enum."E", enum."S"] items=["NW", "N", "NE", "E", "SE", "S", "SW", "W"]
                      n146 = Select(t=w489, s=w490, f=w488) -> (s? t:f=w487:T1[])
                    }
                  }
                }
              }
              n147 = for {
                tunnel: w404 -> [w425] mode=indexing
                tunnel: w396 -> [w428]
                tunnel: [w426] -> w403
                tunnel: [w425] -> w402
                stop <- w426 stop-if-true
                n148 = Index Array(array=w428, index=w425) -> (element=w427:i32)
                n149 = Equal To 0?(x=w427) -> (x = 0?=w426:bool)
              }
              n150 = case shown="False" w403 {
                tunnel: [Action_Enum."Wait" ("Action") Action_Enum."Move" ("Action")] -> w411
                tunnel: w402 -> [_ w422]
                tunnel: w412 -> [w416 w423]
                tunnel: [w415 w421] -> w413
                tunnel: w399 -> [w414 _]
                frame False {
                  n151 = case shown="True" w414 {
                    tunnel: w416 -> [w418 w420]
                    tunnel: [w418 w419] -> w415
                    frame False {
                    }
                    frame True {
                      n152 = call "Increment Stage.vi"("Circle the Wagons in"=w420) -> ("Circle the Wagons out"=w419:refnum<class "Circle the Wagons.lvclass">)  [unwired: 10 in]
                    }
                  }
                }
                frame True {
                  n153 = call "Update Position.vi"("Direction"=w422, "Circle the Wagons in"=w423) -> ("Circle the Wagons out"=w421:refnum<class "Circle the Wagons.lvclass">)  [unwired: 9 in]
                }
              }
            }
            frame 4 {
              # "Replication Ring"
              n154 = Boolean Array To Number(Boolean array=w495) -> (number=w494:u32)
              n155 = Compound Arithmetic op=ADD(w492, w491) -> (w500:i32)
              n156 = Compound Arithmetic op=AND(w500, 1 ("value")) -> (w498:i32)
              n157 = Not Equal To 0?(x=w498) -> (x != 0?=w497:bool)
              n158 = case shown="True" w497 {
                tunnel: w503 -> [w507 w531]
                tunnel: w494 -> [w511 w537]
                tunnel: w496 -> [w512 w536]
                tunnel: [w509 w532] -> w501
                tunnel: [w507 w529] -> w504
                tunnel: [w505 w530] -> w502
                tunnel: [w508 _] -> w493
                tunnel: w492 -> [_ w528]
                tunnel: w491 -> [_ w527]
                frame False {
                  n159 = case shown="9" w511 {
                    tunnel: [_ w522 w523 w524 w525 w526 _] -> w506
                    frame 9 {
                    }
                    frame 1 {
                      w522 = T1[] [enum."E"] items=["NW", "N", "NE", "E", "SE", "S", "SW", "W"]
                    }
                    frame 2, 3 {
                      w523 = T1[] [enum."S"] items=["NW", "N", "NE", "E", "SE", "S", "SW", "W"]
                    }
                    frame 6 {
                      w524 = T1[] [enum."NW"] items=["NW", "N", "NE", "E", "SE", "S", "SW", "W"]
                    }
                    frame 4, 12 {
                      w525 = T1[] [enum."E"] items=["NW", "N", "NE", "E", "SE", "S", "SW", "W"]
                    }
                    frame 8 {
                      w526 = T1[] [enum."S"] items=["NW", "N", "NE", "E", "SE", "S", "SW", "W"]
                    }
                    frame Default {
                    }
                  }
                  n160 = for {
                    tunnel: w512 -> [w516]
                    tunnel: [w514] -> w510
                    tunnel: w506 -> [w513] mode=indexing
                    tunnel: [w513] -> w505
                    stop <- w514 stop-if-true
                    n161 = Index Array(array=w516, index=w513) -> (element=w515:i32)
                    n162 = Equal To 0?(x=w515) -> (x = 0?=w514:bool)
                  }
                  n163 = case shown="True" w510 {
                    tunnel: [Action_Enum."Wait" ("Action") Action_Enum."Replicate" ("Action")] -> w509
                    tunnel: [_ w520] -> w508
                    tunnel: w507 -> [_ w519]
                    tunnel: w505 -> [_ w518]
                    frame False {
                    }
                    frame True {
                      n164 = call "Update Position.vi"("Direction"=w518, "Circle the Wagons in"=w519) -> ("Circle the Wagons out"=w520:refnum<class "Circle the Wagons.lvclass">)  [unwired: 9 in]
                    }
                  }
                }
                frame True {
                  n165 = case shown="1" w537 {
                    tunnel: [_ w554 w560 w562 w564 w566 w568 w571] -> w534
                    tunnel: [_ w553 w559 w561 w563 w565 w567 w570] -> w535
                    tunnel: w528 -> [_ w552 _ _ _ _ _ _]
                    tunnel: w527 -> [_ _ _ _ _ _ _ w569]
                    frame Default {
                    }
                    frame 1 {
                      n166 = case shown="3" w552 {
                        tunnel: [w556 w558] -> w554
                        tunnel: [w555 w557] -> w553
                        frame 3 {
                          w555 = T1[] [enum."N", enum."NE"] items=["NW", "N", "NE", "E", "SE", "S", "SW", "W"]
                          w556 = T1[] [enum."N", enum."NE"] items=["NW", "N", "NE", "E", "SE", "S", "SW", "W"]
                        }
                        frame Default {
                          w557 = T1[] [enum."NW", enum."N"] items=["NW", "N", "NE", "E", "SE", "S", "SW", "W"]
                          w558 = T1[] [enum."N", enum."NE"] items=["NW", "N", "NE", "E", "SE", "S", "SW", "W"]
                        }
                      }
                    }
                    frame 3 {
                      w559 = T1[] [enum."NW", enum."N", enum."NE", enum."E"] items=["NW", "N", "NE", "E", "SE", "S", "SW", "W"]
                      w560 = T1[] [enum."N", enum."NE", enum."E", enum."SE"] items=["NW", "N", "NE", "E", "SE", "S", "SW", "W"]
                    }
                    frame 2 {
                      w561 = T1[] [enum."NE", enum."E"] items=["NW", "N", "NE", "E", "SE", "S", "SW", "W"]
                      w562 = T1[] [enum."E", enum."SE"] items=["NW", "N", "NE", "E", "SE", "S", "SW", "W"]
                    }
                    frame 6 {
                      w563 = T1[] [enum."NW", enum."S"] items=["NW", "N", "NE", "E", "SE", "S", "SW", "W"]
                      w564 = T1[] [enum."NW", enum."SW"] items=["NW", "N", "NE", "E", "SE", "S", "SW", "W"]
                    }
                    frame 4 {
                      w565 = T1[] [enum."SW", enum."S"] items=["NW", "N", "NE", "E", "SE", "S", "SW", "W"]
                      w566 = T1[] [enum."S", enum."SE"] items=["NW", "N", "NE", "E", "SE", "S", "SW", "W"]
                    }
                    frame 12 {
                      w567 = T1[] [enum."NW", enum."W", enum."SW", enum."S"] items=["NW", "N", "NE", "E", "SE", "S", "SW", "W"]
                      w568 = T1[] [enum."W", enum."SW", enum."S", enum."SE"] items=["NW", "N", "NE", "E", "SE", "S", "SW", "W"]
                    }
                    frame 8 {
                      n167 = case shown="3" w569 {
                        tunnel: [w573 w575] -> w571
                        tunnel: [w572 w574] -> w570
                        frame 3 {
                          w572 = T1[] [enum."W", enum."SW"] items=["NW", "N", "NE", "E", "SE", "S", "SW", "W"]
                          w573 = T1[] [enum."W", enum."SW"] items=["NW", "N", "NE", "E", "SE", "S", "SW", "W"]
                        }
                        frame Default {
                          w574 = T1[] [enum."NW", enum."W"] items=["NW", "N", "NE", "E", "SE", "S", "SW", "W"]
                          w575 = T1[] [enum."W", enum."SW"] items=["NW", "N", "NE", "E", "SE", "S", "SW", "W"]
                        }
                      }
                    }
                  }
                  n168 = for {
                    tunnel: w536 -> [w550]
                    tunnel: w535 -> [w551] mode=indexing
                    tunnel: w534 -> [w544] mode=indexing
                    tunnel: [w545] -> w533
                    tunnel: [w544] -> w530
                    stop <- w545 stop-if-true
                    n169 = Index Array(array=w550, index=w551) -> (element=w549:i32)
                    n170 = Index Array(array=w550, index=w544) -> (element=w548:i32)
                    n171 = Equal To 0?(x=w549) -> (x = 0?=w547:bool)
                    n172 = Equal To 0?(x=w548) -> (x = 0?=w546:bool)
                    n173 = Compound Arithmetic op=AND(w547, w546) -> (w545:bool)
                  }
                  n174 = case shown="True" w533 {
                    tunnel: [Action_Enum."Wait" ("Action") Action_Enum."Move" ("Action")] -> w532
                    tunnel: w531 -> [w538 w542]
                    tunnel: w530 -> [_ w541]
                    tunnel: [w538 w540] -> w529
                    frame False {
                    }
                    frame True {
                      n175 = call "Update Position.vi"("Direction"=w541, "Circle the Wagons in"=w542) -> ("Circle the Wagons out"=w540:refnum<class "Circle the Wagons.lvclass">)  [unwired: 9 in]
                    }
                  }
                }
              }
            }
            frame Default {
              # "Inner Ring"
              n176 = Less?(x=w577, y=w576) -> (x < y?=w578:bool)
              n177 = case shown="False" w578 {
                tunnel: [w589 w618] -> w581
                tunnel: w580 -> [w588 w617]
                tunnel: [w587 w616] -> w579
                tunnel: w577 -> [w586 w615]
                tunnel: w576 -> [w585 w614]
                frame True {
                  n178 = case shown="4" w586 {
                    tunnel: [w596 w600 w611] -> w589
                    tunnel: w588 -> [w594 w601 w612]
                    tunnel: [w590 w599 w610] -> w587
                    tunnel: w585 -> [_ w598 _]
                    frame 4 {
                      w596 = Direction_Enum."W" ("Direction")
                      n179 = Index Array(array=w594, index=Direction_Enum."SW" ("Direction")) -> (element=w595:i32)
                      n180 = Index Array(array=w594, index=w596) -> (element=w597:i32)
                      n181 = Equal To 0?(x=w595) -> (x = 0?=w591:bool)
                      n182 = Equal To 0?(x=w597) -> (x = 0?=w592:bool)
                      n183 = Compound Arithmetic op=AND(w592, w591) -> (w590:bool)
                    }
                    frame 3 {
                      n184 = case shown="4" w598 {
                        tunnel: w601 -> [w604 w608]
                        tunnel: [w603 w606] -> w600
                        tunnel: [w602 w607] -> w599
                        frame Default {
                          w603 = Direction_Enum."N" ("Direction")
                          n185 = Index Array(array=w604, index=w603) -> (element=w605:i32)
                          n186 = Equal To 0?(x=w605) -> (x = 0?=w602:bool)
                        }
                        frame 4 {
                          w606 = Direction_Enum."NW" ("f")
                          n187 = Index Array(array=w608, index=w606) -> (element=w609:i32)
                          n188 = Equal To 0?(x=w609) -> (x = 0?=w607:bool)
                        }
                      }
                    }
                    frame Default {
                      w611 = Direction_Enum."NW" ("Direction")
                      n189 = Index Array(array=w612, index=w611) -> (element=w613:i32)
                      n190 = Equal To 0?(x=w613) -> (x = 0?=w610:bool)
                    }
                  }
                }
                frame False {
                  n191 = case shown="3" w614 {
                    tunnel: [w625 w629 w640] -> w618
                    tunnel: w617 -> [w623 w630 w641]
                    tunnel: [w619 w628 w639] -> w616
                    tunnel: w615 -> [_ w627 _]
                    frame 4 {
                      w625 = Direction_Enum."N" ("Direction")
                      n192 = Index Array(array=w623, index=Direction_Enum."NE" ("Direction")) -> (element=w624:i32)
                      n193 = Index Array(array=w623, index=w625) -> (element=w626:i32)
                      n194 = Equal To 0?(x=w624) -> (x = 0?=w620:bool)
                      n195 = Equal To 0?(x=w626) -> (x = 0?=w621:bool)
                      n196 = Compound Arithmetic op=AND(w621, w620) -> (w619:bool)
                    }
                    frame 3 {
                      n197 = case shown="4" w627 {
                        tunnel: w630 -> [w633 w637]
                        tunnel: [w632 w635] -> w629
                        tunnel: [w631 w636] -> w628
                        frame Default {
                          w632 = Direction_Enum."W" ("Direction")
                          n198 = Index Array(array=w633, index=w632) -> (element=w634:i32)
                          n199 = Equal To 0?(x=w634) -> (x = 0?=w631:bool)
                        }
                        frame 4 {
                          w635 = Direction_Enum."NW" ("f")
                          n200 = Index Array(array=w637, index=w635) -> (element=w638:i32)
                          n201 = Equal To 0?(x=w638) -> (x = 0?=w636:bool)
                        }
                      }
                    }
                    frame Default {
                      w640 = Direction_Enum."NW" ("Direction")
                      n202 = Index Array(array=w641, index=w640) -> (element=w642:i32)
                      n203 = Equal To 0?(x=w642) -> (x = 0?=w639:bool)
                    }
                  }
                }
              }
              n204 = case shown="True" w579 {
                tunnel: [Action_Enum."Wait" ("Action") Action_Enum."Move" ("Action")] -> w583
                tunnel: [w643 w647] -> w582
                tunnel: w584 -> [w643 w648]
                tunnel: w581 -> [_ w646]
                frame False {
                }
                frame True {
                  n205 = call "Update Position.vi"("Direction"=w646, "Circle the Wagons in"=w648) -> ("Circle the Wagons out"=w647:refnum<class "Circle the Wagons.lvclass">)  [unwired: 9 in]
                }
              }
            }
          }
        }
      }
    }
  }
  "Runner out" <- w12
  "Action" <- w7
  "Direction" <- w8
  "Replicated" <- w6
  "error out" <- "error in (no error)"
